vi "Create Valve.vi"(5 "Group":refnum<class "Group.lvclass">, 8 "error in (no error)":errorcluster, 10 "Config Element":refnum<class "Config Element.lvclass">, 11 "ValveControlModule in":refnum<class "DigitalControlModule.lvclass">) -> (0 "error out":errorcluster, 3 "ValveControlModule out":refnum<class "DigitalControlModule.lvclass">)   [LabVIEW 2020, in "VolatusControl.lvlib" / "DigitalControlModule.lvclass"]
uses:
  DigitalControlModule.lvclass
  DigitalControlModule.lvclass/DigitalControlModule.ctl
  lv-cdm/CDM-Config/Config Element/Config Element.lvclass
  Volatus/Module/Module.lvclass
  VolatusConfig/VolatusConfig.lvlib
  VolatusConfig/Meta Type.ctl
  DigitalControl/DigitalControl.lvclass
  C:/dev/lv20CE/relink/lv-volatus/Volatus/Module/Module.lvclass
  C:/dev/lv20CE/relink/lv-volatus/VolatusControl/DigitalControlModule/DigitalControlModule.lvclass
  lv-vecto/Vecto/Group/Group.lvclass
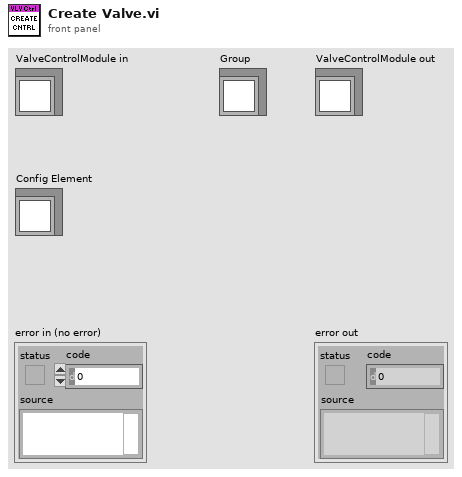
[diagram p1: front panel]
types:
  T1 = typedef "VolatusConfig.lvlib/Meta Type.ctl" = enum16{"UNKNOWN", "VL_System", "VL_Cluster", "VL_Node", "VL_Task", "VL_Group", "VL_Channel", "VL_Task_List", "VL_Scaling", "VL_Sensor", "VL_Sensor_List", "VL_Scale"}
  T2 = map{string, refnum<class "DigitalControl.lvclass">}
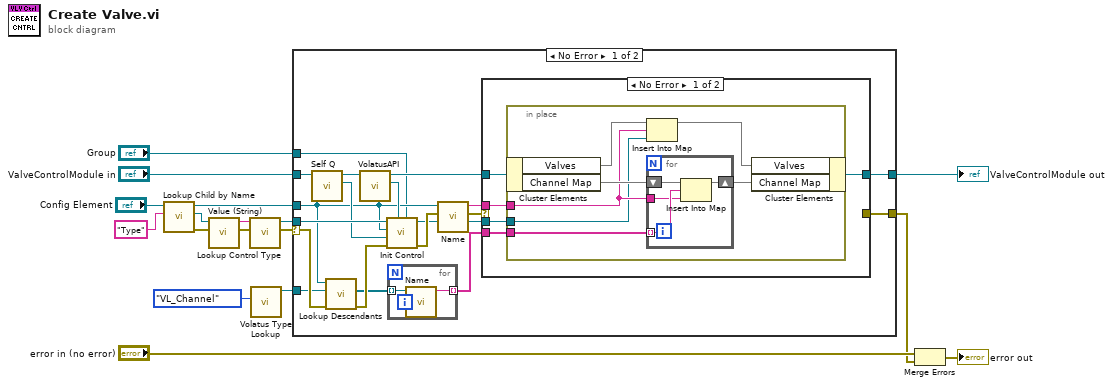
[diagram p0: block diagram]
diagram:
  n1 = call "Lookup Child by Name.vi"("Name"="Type", "Config Element in"="Config Element") -> ("error out"=w12:errorcluster, "Child"=w13:refnum<class "Config Element.lvclass">, "Config Element out"=w7:refnum<class "Config Element.lvclass">)  [unwired: 6 in, 1 out]
  n2 = call "Value (String).vi"("error in (no error)"=w12, "Config Element in"=w13) -> ("error out"=w10:errorcluster, "String Value"=w11:string)  [unwired: 8 in]
  n3 = call "Lookup Control Type.vi"("error in (no error)"=w10, "Control Type"=w11) -> ("error out"=w6:errorcluster, "ValveControl"=w9:refnum<class "DigitalControl.lvclass">)  [unwired: 8 in]
  n4 = call "Volatus Type Lookup.vi"("Meta Type"=Meta_Type."VL_Channel") -> ("Config Lookup out"=w4:refnum<class "Config Lookup.lvclass">)  [unwired: 9 in, 1 out]
  n5 = case shown="No Error" w6 {
    selector: w6 -> [w36 w57]
    tunnel: "ValveControlModule in" -> [w35 w58]
    tunnel: w9 -> [w34 _]
    tunnel: [w21 w58] -> w8
    tunnel: w7 -> [w28 _]
    tunnel: w4 -> [w30 _]
    tunnel: [w19 w57] -> w2
    tunnel: "Group" -> [w18 _]
    frame No Error {
      n6 = call "Self Q.vi"("Module in"=w35) -> ("Self Q"=w31:refnum<class "MessageQ.lvclass">, "Module out"=w32:refnum<class "DigitalControlModule.lvclass">)  [unwired: 9 in]
      n7 = call "Lookup Descendants.vi"("error in (no error)"=w36, "Lookup"=w30, "Config Element in"=w28) -> ("error out"=w29:errorcluster, "Descendants"=w26:refnum<class "Config Element.lvclass">[])  [unwired: 6 in, 1 out]
      n8 = call "VolatusAPI.vi"("Module in"=w32) -> ("VolatusAPI"=w33:refnum<class "VolatusAPI.lvclass">, "Module out"=w25:refnum<class "DigitalControlModule.lvclass">)  [unwired: 9 in]
      n9 = call-dynamic "Init Control.vi"("Group"=w18, "VolatusAPI"=w33, "error in (no error)"=w29, "Control MsgQ"=w31, "Config Element"=w28, "Valve in"=w34) -> ("error out"=w27:errorcluster, "Valve out"=w22:refnum<class "DigitalControl.lvclass">)  [unwired: 4 in]
      n10 = for {
        tunnel: w26 -> [w56] mode=indexing
        tunnel: [w55] -> w23 mode=indexing
        n11 = call "Name.vi"("Config Element in"=w56) -> ("Name"=w55:string)  [unwired: 9 in, 1 out]
      }
      n12 = call "Name.vi"("error in (no error)"=w27, "Config Element in"=w28) -> ("error out"=w20:errorcluster, "Name"=w24:string)  [unwired: 8 in]
      n13 = case shown="No Error" w20 {
        selector: w20 -> [_ w54]
        tunnel: w25 -> [w41 w53]
        tunnel: w24 -> [w40 _]
        tunnel: w23 -> [w39 _]
        tunnel: w22 -> [w38 _]
        tunnel: [w37 w53] -> w21
        tunnel: [_ w54] -> w19
        frame No Error {
          n14 = in-place {
            in-place-border: w40 -> [w45]
            in-place-border: w39 -> [w44]
            in-place-border: w38 -> [w42]
            n15 = in-place-cluster #1(w41) -> ("Valves"=w48:T2, "Channel Map"=w46:map{string, string})
            n16 = Insert Into Map(map in=w48, key=w45, value=w42) -> (map out=w47:T2)  [unwired: 2 out]
            n17 = for {
              shift-right: [w49] -> w43
              shift-left: w46 -> [w52]
              tunnel: w45 -> [w50]
              tunnel: w44 -> [w51] mode=indexing
              n18 = Insert Into Map(map in=w52, key=w51, value=w50) -> (map out=w49:map{string, string})  [unwired: 2 out]
            }
            n19 = in-place-cluster #1("Valves"=w47, "Channel Map"=w43) -> (w37:refnum<class "DigitalControlModule.lvclass">)
          }
        }
        frame Error {
        }
      }
    }
    frame Error {
    }
  }
  "ValveControlModule out" <- w8
  n20 = Merge Errors("error in (no error)", w2) -> (→"error out":errorcluster)
